vi "CHANGE_ITEM2STOCK.vi"(4 "date (to)":timestamp, 6 "date (From)":timestamp, 7 "connection reference":T1, 9 "DATABASE":string, 10 "data":T2[](array[typedef]), 11 "Output Type":string) -> (3 "Table Out":string[][](array[string]))   [LabVIEW 2015]
uses:
  Controls/ITEM_CODE_CLUSTER.ctl
  <vilib>/addons/database/Connection.llb/Conn ObjectReference.ctl
  <vilib>/addons/database/_DB Variant To Data/Database Variant To Data.xnode
  <vilib>/addons/database/NI_Database_API.lvlib
panel:
  in  "Data type":T2[](array[typedef])
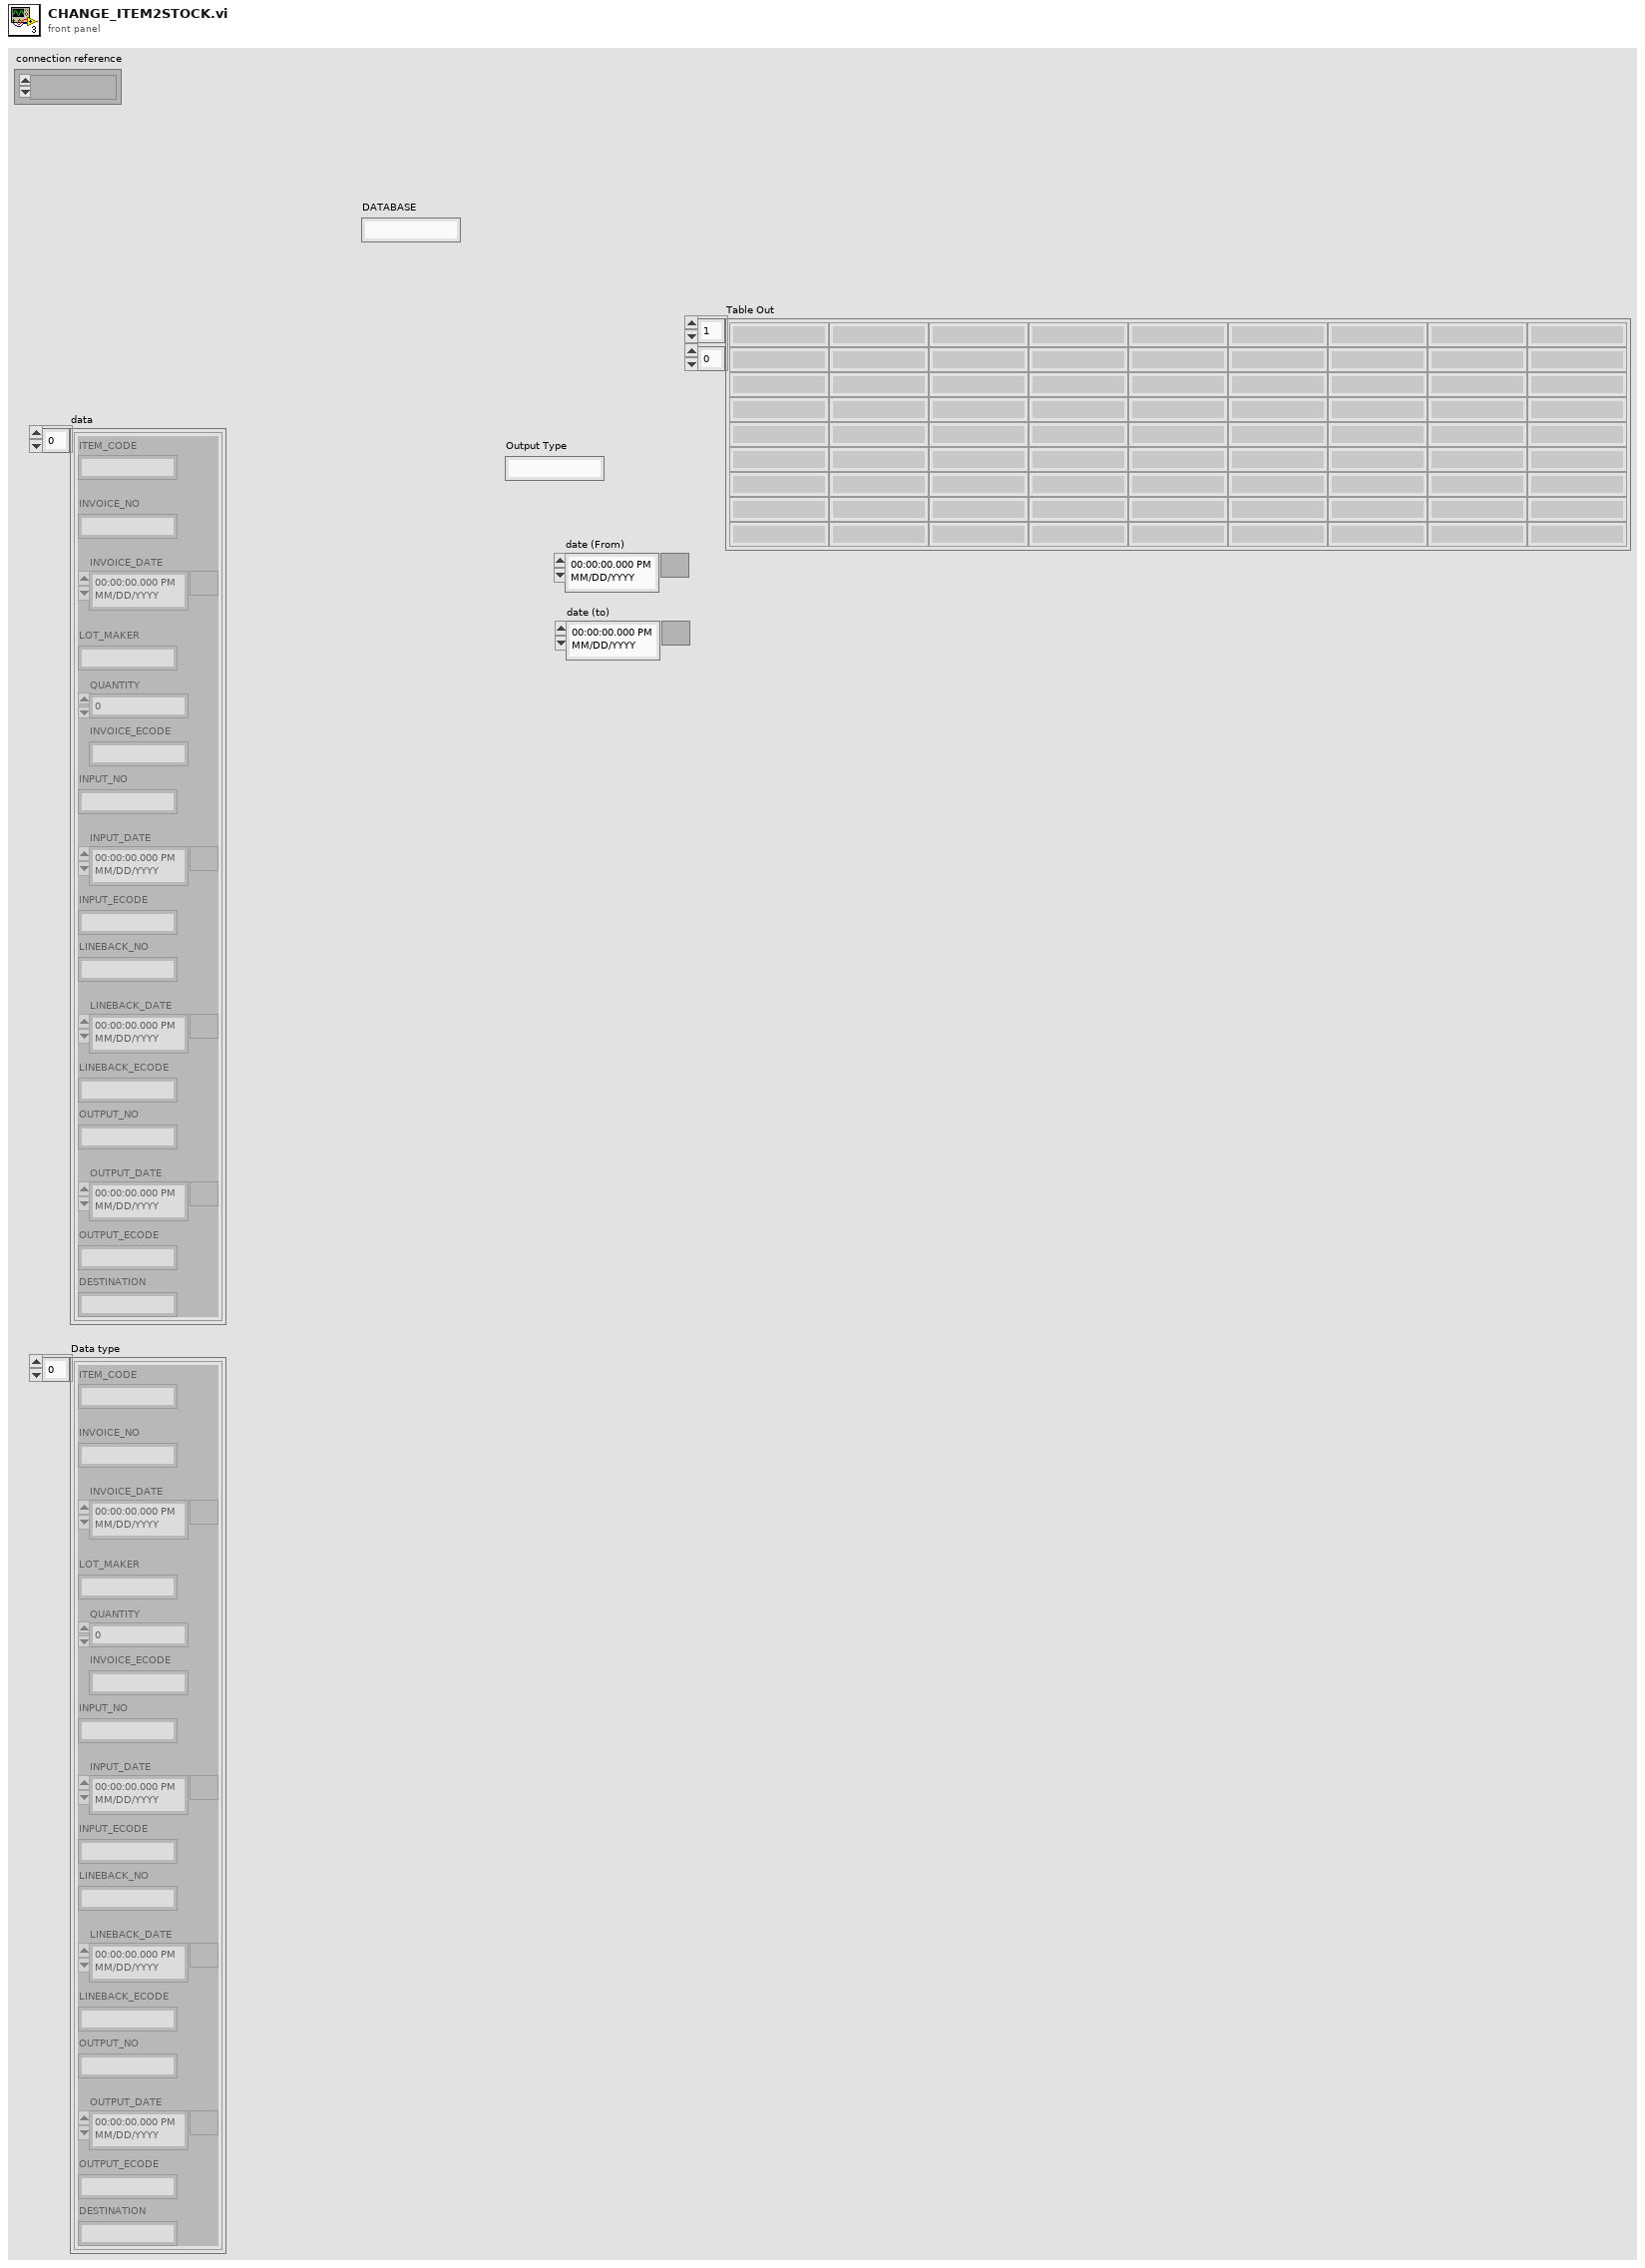
[diagram p1: front panel]
types:
  T1 = typedef "NI_Database_API.lvlib/Conn ObjectReference.ctl" = refnum<k1>
  T2 = typedef "ITEM_CODE_CLUSTER.ctl" = cluster{"ITEM_CODE":string, "INVOICE_NO":string, "INVOICE_DATE":timestamp, "LOT_MAKER":string, "QUANTITY":dbl, "INVOICE_ECODE":string, "INPUT_NO":string, "INPUT_DATE":timestamp, "INPUT_ECODE":string, "LINEBACK_NO":string, "LINEBACK_DATE":timestamp, "LINEBACK_ECODE":string, "OUTPUT_NO":string, "OUTPUT_DATE":timestamp, "OUTPUT_ECODE":string, "DESTINATION":string}
  T3 = cluster{"OUTPUT_DATE":timestamp, "Input":dbl, "Lineback":dbl, "QUANTITY":dbl, "Inline":dbl, "INVOICE_NO":string, "PO":string, "DESTINATION":string, "Stock":dbl, "Line Stock":dbl, "OUTPUT_ECODE":string, "PO":string}[]
  T4 = cluster{"LINEBACK_DATE":timestamp, "Input":dbl, "QUANTITY":dbl, "output":dbl, "Inline":dbl, "INVOICE_NO":string, "PO":string, "LINEBACK_NO":string, "Stock":dbl, "Line Stock":dbl, "LINEBACK_ECODE":string, "PO":string}[]
  T5 = cluster{"INPUT_DATE":timestamp, "QUANTITY":dbl, "Lineback":dbl, "output":dbl, "Inline":dbl, "INVOICE_NO":string, "PO":string, "Lot":string, "Stock":dbl, "Line Stock":dbl, "INPUT_ECODE":string, "INPUT_NO":string}[]
  T6 = cluster{"LINEBACK_DATE":timestamp, "Input":dbl, "QUANTITY":dbl, "output":dbl, "Inline":dbl, "INVOICE_NO":string, "PO":string, "LINEBACK_NO":string, "Stock":dbl, "Line Stock":dbl, "LINEBACK_ECODE":string, "PO":string}
  T7 = cluster{"OUTPUT_DATE":timestamp, "Input":dbl, "Lineback":dbl, "QUANTITY":dbl, "Inline":dbl, "INVOICE_NO":string, "OUTPUT_NO":string, "result string":string, "Stock":dbl, "Line Stock":dbl, "OUTPUT_ECODE":string, "PO":string}
  T8 = cluster{"INPUT_DATE":timestamp, "QUANTITY":dbl, "Lineback":dbl, "output":dbl, "Inline":dbl, "INVOICE_NO":string, "INPUT_NO":string, "Lot":string, "Stock":dbl, "Line Stock":dbl, "INPUT_ECODE":string, "INPUT_NO":string}
  T9 = cluster{"date (From)":timestamp, "input_initail":dbl, "line back initail":dbl, "output initail":dbl, "Inline":dbl, "PO":string, "PO":string, "PO":string, "Stock":dbl, "Line Stock":dbl, "PO":string, "PO":string}
  T10 = cluster{"INPUT_DATE":timestamp, "QUANTITY":dbl, "Lineback":dbl, "output":dbl, "Inline":dbl, "INVOICE_NO":string, "PO":string, "Lot":string, "Stock":dbl, "Line Stock":dbl, "INPUT_ECODE":string, "INPUT_NO":string}
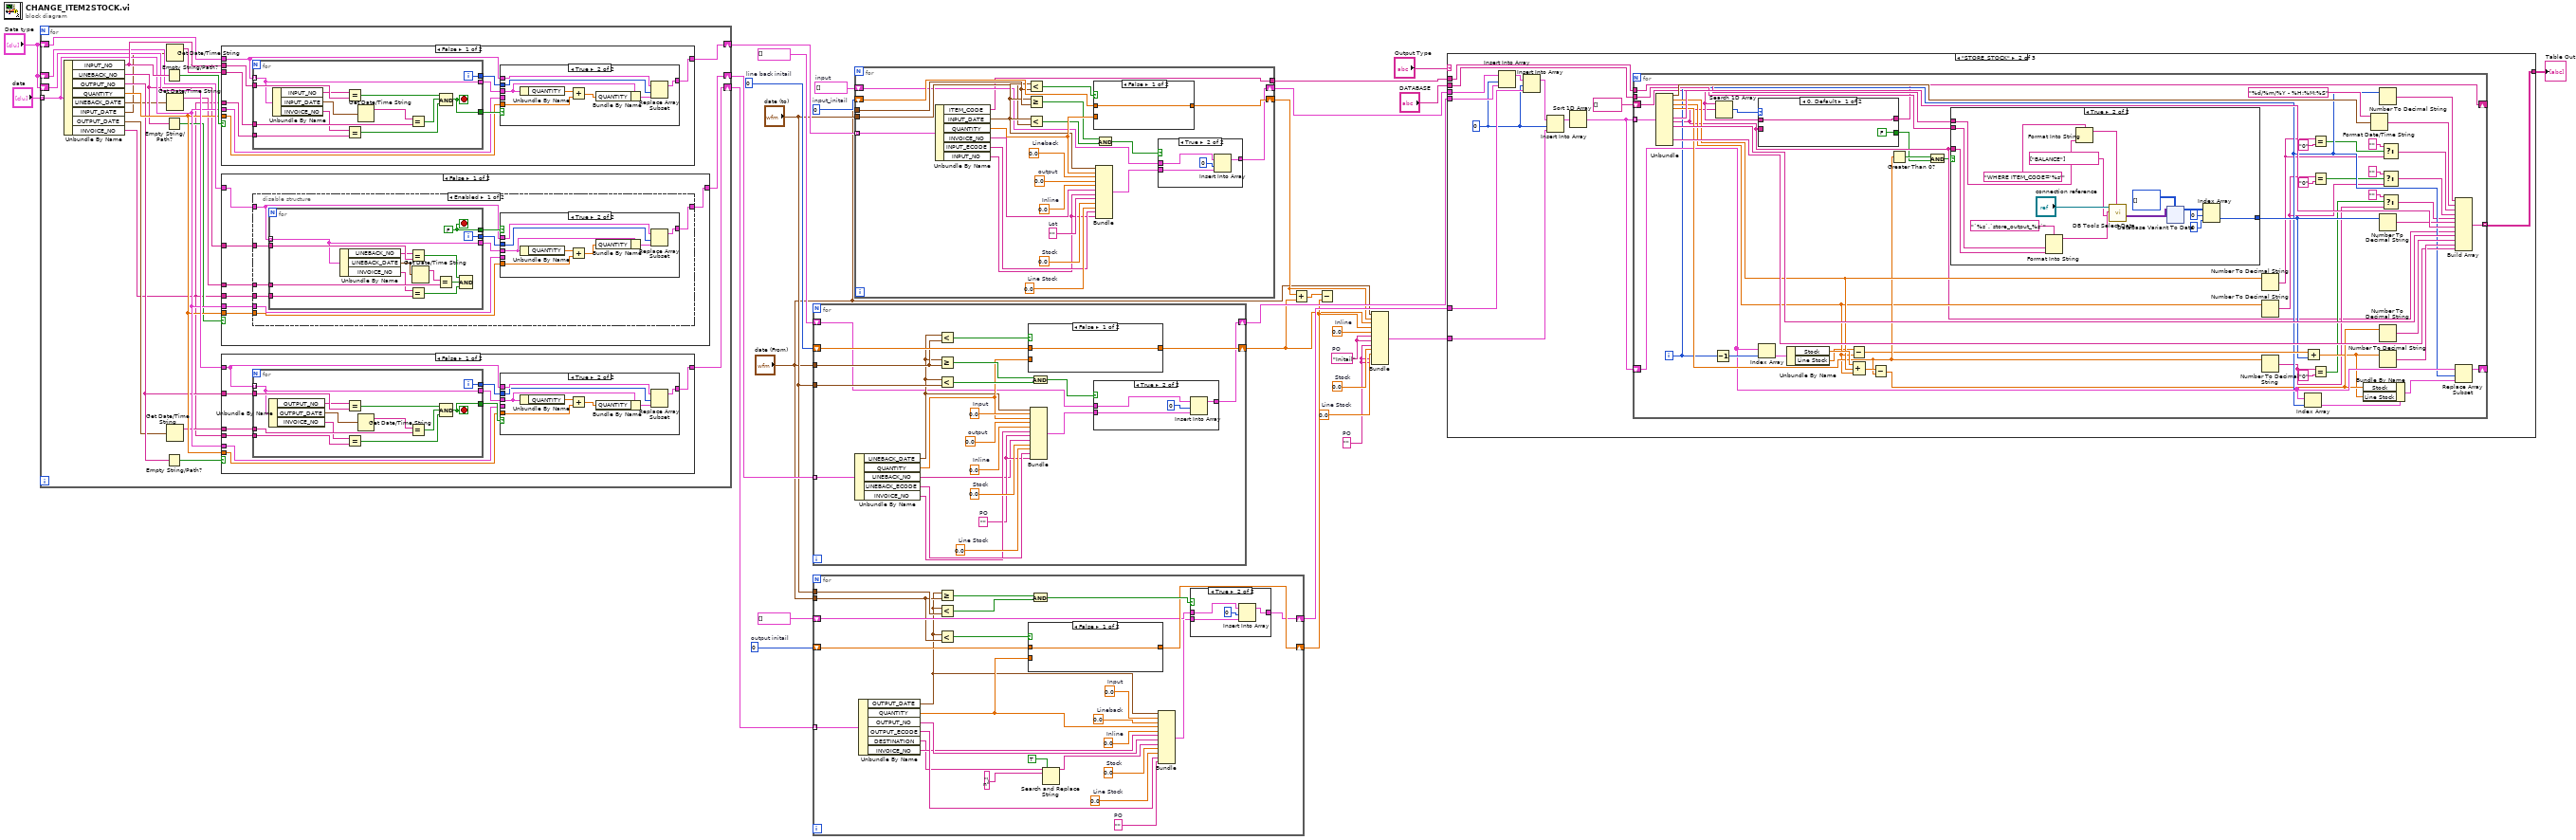
[diagram p0: block diagram]
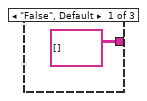
[diagram p2: hidden frame]
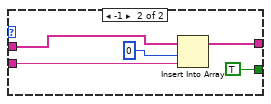
[diagram p3: hidden frame]
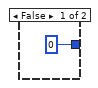
[diagram p4: hidden frame]
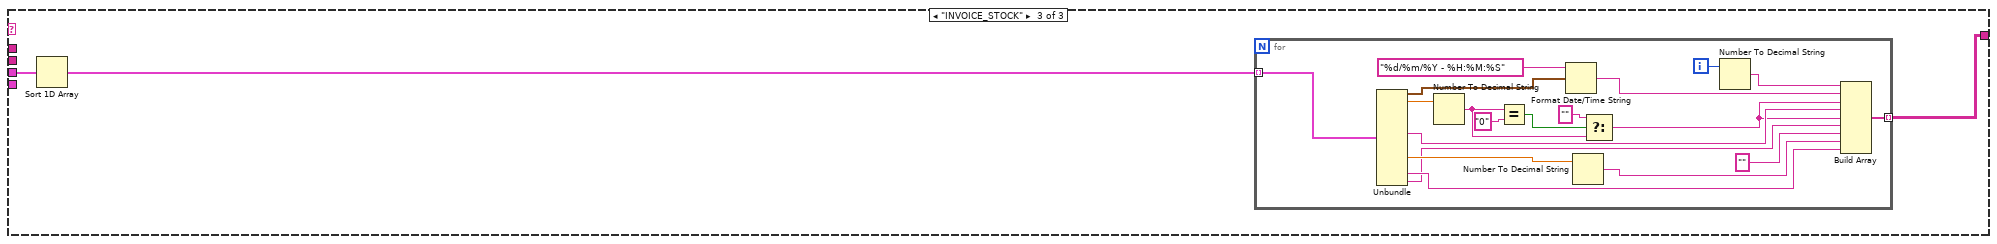
[diagram p5: hidden frame]
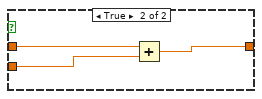
[diagram p7: hidden frame]
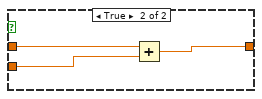
[diagram p9: hidden frame]
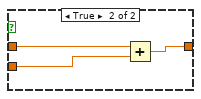
[diagram p11: hidden frame]
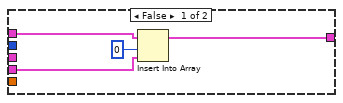
[diagram p12: hidden frame]
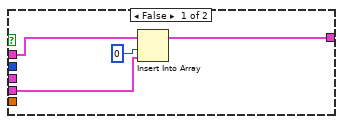
[diagram p14: hidden frame]
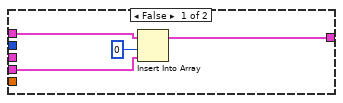
[diagram p17: hidden frame]
diagram:
  w5 = "Initail"  # PO
  w12 = 0.0  # Line Stock
  w11 = 0.0  # Stock
  w4 = ""  # PO
  w6 = 0.0  # Inline
  w17 = 0  # output initail
  w19 = 0  # line back initail
  w22 = T5 []  # input
  w23 = 0  # input_initail
  n1 = for {
    shift-right: [w48] -> w28
    shift-left: "Data type" -> [w51]
    shift-right: [w46] -> w29
    shift-left: "Data type" -> [w47]
    shift-right: [w44] -> w30
    shift-left: "Data type" -> [w45]
    tunnel: "data" -> [w43] mode=indexing
    n2 = Unbundle By Name(w43) -> ("INPUT_NO"=w50:string, "LINEBACK_NO"=w41:string, "OUTPUT_NO"=w39:string, "QUANTITY"=w42:dbl, "LINEBACK_DATE"=w37:timestamp, "INPUT_DATE"=w35:timestamp, "OUTPUT_DATE"=w33:timestamp, "INVOICE_NO"=w31:string)
    n3 = Empty String/Path?(string/path=w50) -> (empty?=w49:bool)
    n4 = Empty String/Path?(string/path=w41) -> (empty?=w40:bool)
    n5 = Empty String/Path?(string/path=w39) -> (empty?=w38:bool)
    n6 = Get Date/Time String(seconds (now)=w35) -> (date string=w34:string)  [unwired: 2 in, 1 out]
    n7 = Get Date/Time String(seconds (now)=w37) -> (date string=w36:string)  [unwired: 2 in, 1 out]
    n8 = Get Date/Time String(seconds (now)=w33) -> (date string=w32:string)  [unwired: 2 in, 1 out]
    n9 = case shown="False" w49 {
      tunnel: w51 -> [w138 w167]
      tunnel: w50 -> [w140 _]
      tunnel: w42 -> [w136 _]
      tunnel: [w135 w167] -> w48
      tunnel: w43 -> [w134 _]
      tunnel: w34 -> [w133 _]
      tunnel: w31 -> [w132 _]
      frame False {
        n10 = for {
          tunnel: w138 -> [w163] mode=indexing
          tunnel: w140 -> [w166]
          tunnel: [w157] -> w141
          tunnel: [w164] -> w139
          tunnel: [w163] -> w137
          tunnel: w133 -> [w162]
          tunnel: w132 -> [w156]
          i -> [w164]
          stop <- w157 stop-if-true
          n11 = Unbundle By Name(w163) -> ("INPUT_NO"=w165:string, "INPUT_DATE"=w161:timestamp, "INVOICE_NO"=w155:string)
          n12 = Equal?(x=w165, y=w166) -> (x = y?=w159:bool)
          n13 = Equal?(x=w155, y=w156) -> (x = y?=w154:bool)
          n14 = Get Date/Time String(seconds (now)=w161) -> (date string=w160:string)  [unwired: 2 in, 1 out]
          n15 = Equal?(x=w160, y=w162) -> (x = y?=w158:bool)
          n16 = Compound Arithmetic op=AND(w159, w158, w154) -> (w157:bool)
        }
        n17 = case shown="True" w141 {
          tunnel: w139 -> [_ w152]
          tunnel: w138 -> [w145 w153]
          tunnel: w137 -> [_ w150]
          tunnel: w136 -> [_ w148]
          tunnel: [w142 w147] -> w135
          tunnel: w134 -> [w144 _]
          frame False {
            n18 = Insert Into Array(array=w145, index=0, new element=w144) -> (w142:T2[])
          }
          frame True {
            n19 = Unbundle By Name(w150) -> ("QUANTITY"=w151:dbl)
            n20 = Add(x=w151, y=w148) -> (x+y=w149:dbl)
            n21 = Bundle By Name(cluster=w150, "QUANTITY"=w149) -> (w146:T2)
            n22 = Replace Array Subset(array=w153, new element=w146, index=w152) -> (w147:T2[])
          }
        }
      }
      frame True {
      }
    }
    n23 = case shown="False" w40 {
      tunnel: w47 -> [w93 w131]
      tunnel: w41 -> [w94 _]
      tunnel: w42 -> [w92 _]
      tunnel: [w91 w131] -> w46
      tunnel: w43 -> [w90 _]
      tunnel: w36 -> [w89 _]
      tunnel: w31 -> [w88 _]
      frame False {
        n24 = disable-structure shown="Enabled" {
          disable-tunnel: w94 -> [w103 _]
          disable-tunnel: w93 -> [w101 w130]
          disable-tunnel: w92 -> [w99 _]
          disable-tunnel: [w98 w130] -> w91
          disable-tunnel: w90 -> [w97 _]
          disable-tunnel: w89 -> [w96 _]
          disable-tunnel: w88 -> [w95 _]
          frame Enabled {
            n25 = for {
              tunnel: w101 -> [w126] mode=indexing
              tunnel: w103 -> [w129]
              tunnel: [w120] -> w104
              tunnel: [w127] -> w102
              tunnel: [w126] -> w100
              tunnel: w96 -> [w125]
              tunnel: w95 -> [w118]
              i -> [w127]
              stop <- w120 stop-if-true
              w120 = FALSE
              n26 = Unbundle By Name(w126) -> ("LINEBACK_NO"=w128:string, "LINEBACK_DATE"=w124:timestamp, "INVOICE_NO"=w119:string)
              n27 = Equal?(x=w128, y=w129) -> (x = y?=w122:bool)
              n28 = Equal?(x=w119, y=w118) -> (x = y?=w117:bool)
              n29 = Get Date/Time String(seconds (now)=w124) -> (date string=w123:string)  [unwired: 2 in, 1 out]
              n30 = Equal?(x=w123, y=w125) -> (x = y?=w121:bool)
              n31 = Compound Arithmetic op=AND(w122, w121, w117) -> ()  [unwired: 1 out]
            }
            n32 = case shown="True" w104 {
              tunnel: w102 -> [_ w115]
              tunnel: w101 -> [w108 w116]
              tunnel: w100 -> [_ w113]
              tunnel: w99 -> [_ w111]
              tunnel: [w105 w110] -> w98
              tunnel: w97 -> [w107 _]
              frame False {
                n33 = Insert Into Array(array=w108, index=0, new element=w107) -> (w105:T2[])
              }
              frame True {
                n34 = Unbundle By Name(w113) -> ("QUANTITY"=w114:dbl)
                n35 = Add(x=w114, y=w111) -> (x+y=w112:dbl)
                n36 = Bundle By Name(cluster=w113, "QUANTITY"=w112) -> (w109:T2)
                n37 = Replace Array Subset(array=w116, new element=w109, index=w115) -> (w110:T2[])
              }
            }
          }
          frame Disabled {
          }
        }
      }
      frame True {
      }
    }
    n38 = case shown="False" w38 {
      tunnel: w45 -> [w58 w87]
      tunnel: w39 -> [w60 _]
      tunnel: w42 -> [w56 _]
      tunnel: [w55 w87] -> w44
      tunnel: w43 -> [w54 _]
      tunnel: w32 -> [w53 _]
      tunnel: w31 -> [w52 _]
      frame False {
        n39 = for {
          tunnel: w58 -> [w83] mode=indexing
          tunnel: w60 -> [w86]
          tunnel: [w77] -> w61
          tunnel: [w84] -> w59
          tunnel: [w83] -> w57
          tunnel: w53 -> [w80]
          tunnel: w52 -> [w75]
          i -> [w84]
          stop <- w77 stop-if-true
          n40 = Unbundle By Name(w83) -> ("OUTPUT_NO"=w85:string, "OUTPUT_DATE"=w81:timestamp, "INVOICE_NO"=w76:string)
          n41 = Equal?(x=w85, y=w86) -> (x = y?=w79:bool)
          n42 = Equal?(x=w76, y=w75) -> (x = y?=w74:bool)
          n43 = Get Date/Time String(seconds (now)=w81) -> (date string=w82:string)  [unwired: 2 in, 1 out]
          n44 = Equal?(x=w82, y=w80) -> (x = y?=w78:bool)
          n45 = Compound Arithmetic op=AND(w79, w78, w74) -> (w77:bool)
        }
        n46 = case shown="True" w61 {
          tunnel: w59 -> [_ w72]
          tunnel: w58 -> [w65 w73]
          tunnel: w57 -> [_ w70]
          tunnel: w56 -> [_ w68]
          tunnel: [w62 w67] -> w55
          tunnel: w54 -> [w64 _]
          frame False {
            n47 = Insert Into Array(array=w65, index=0, new element=w64) -> (w62:T2[])
          }
          frame True {
            n48 = Unbundle By Name(w70) -> ("QUANTITY"=w71:dbl)
            n49 = Add(x=w71, y=w68) -> (x+y=w69:dbl)
            n50 = Bundle By Name(cluster=w70, "QUANTITY"=w69) -> (w66:T2)
            n51 = Replace Array Subset(array=w73, new element=w66, index=w72) -> (w67:T2[])
          }
        }
      }
      frame True {
      }
    }
  }
  n52 = for {
    tunnel: w29 -> [w190] mode=indexing
    tunnel: "date (From)" -> [w176]
    tunnel: "date (to)" -> [w177]
    shift-right: [w171] -> w18
    shift-left: T4 [] -> [w174]
    shift-right: [w172] -> w8
    shift-left: w19 -> [w179]
    w186 = 0.0  # Line Stock
    w187 = 0.0  # Stock
    w169 = ""  # PO
    w188 = 0.0  # Inline
    w189 = 0.0  # output
    w184 = 0.0  # Input
    n53 = Unbundle By Name(w190) -> ("LINEBACK_DATE"=w175:timestamp, "QUANTITY"=w178:dbl, "LINEBACK_NO"=w168:string, "LINEBACK_ECODE"=w185:string, "INVOICE_NO"=w170:string)
    n54 = Less?(x=w175, y=w176) -> (x < y?=w180:bool)
    n55 = Greater Or Equal?(x=w175, y=w176) -> (x >= y?=w181:bool)
    n56 = Less?(x=w175, y=w177) -> (x < y?=w182:bool)
    n57 = case shown="False" w180 {
      tunnel: w178 -> [_ w198]
      tunnel: w179 -> [w196 w199]
      tunnel: [w196 w197] -> w172
      frame False {
      }
      frame True {
        n58 = Add(x=w199, y=w198) -> (x+y=w197:dbl)
      }
    }
    n59 = Bundle("LINEBACK_DATE"=w175, "Input"=w184, "QUANTITY"=w178, "output"=w189, "Inline"=w188, "INVOICE_NO"=w170, "PO"=w169, "LINEBACK_NO"=w168, "Stock"=w187, "Line Stock"=w186, "LINEBACK_ECODE"=w185, "PO"=w169) -> (w173:T6)  [unwired: 1 in]
    n60 = And(x=w181, y=w182) -> (x .and. y?=w183:bool)
    n61 = case shown="True" w183 {
      tunnel: w174 -> [w191 w195]
      tunnel: w173 -> [_ w193]
      tunnel: [w191 w192] -> w171
      frame False {
      }
      frame True {
        n62 = Insert Into Array(array=w195, index=0, new element=w193) -> (w192:T4)
      }
    }
  }
  n63 = for {
    tunnel: w30 -> [w226] mode=indexing
    shift-right: [w213] -> w9
    shift-left: w17 -> [w215]
    shift-right: [w210] -> w14
    shift-left: T3 [] -> [w212]
    tunnel: "date (to)" -> [w209]
    tunnel: "date (From)" -> [w208]
    w223 = 0.0  # Line Stock
    w224 = 0.0  # Stock
    w205 = ""  # PO
    w225 = 0.0  # Inline
    w220 = 0.0  # Lineback
    w221 = 0.0  # Input
    n64 = Unbundle By Name(w226) -> ("OUTPUT_DATE"=w207:timestamp, "QUANTITY"=w214:dbl, "OUTPUT_NO"=w206:string, "OUTPUT_ECODE"=w222:string, "DESTINATION"=w202:string, "INVOICE_NO"=w204:string)
    n65 = Greater Or Equal?(x=w207, y=w208) -> (x >= y?=w217:bool)
    n66 = Less?(x=w207, y=w209) -> (x < y?=w218:bool)
    n67 = Less?(x=w207, y=w208) -> (x < y?=w216:bool)
    n68 = case shown="False" w216 {
      tunnel: w214 -> [_ w234]
      tunnel: w215 -> [w232 w235]
      tunnel: [w232 w233] -> w213
      frame False {
      }
      frame True {
        n69 = Add(x=w235, y=w234) -> (x+y=w233:dbl)
      }
    }
    n70 = And(x=w217, y=w218) -> (x .and. y?=w219:bool)
    n71 = Search and Replace String(replace all?=TRUE ("replace all? (F)"), input string=w202, search string="\n") -> (result string=w201:string)  [unwired: 5 in, 3 out]
    n72 = Bundle("OUTPUT_DATE"=w207, "Input"=w221, "Lineback"=w220, "QUANTITY"=w214, "Inline"=w225, "INVOICE_NO"=w204, "OUTPUT_NO"=w206, "result string"=w201, "Stock"=w224, "Line Stock"=w223, "OUTPUT_ECODE"=w222, "PO"=w205) -> (w211:T7)  [unwired: 1 in]
    n73 = case shown="True" w219 {
      tunnel: w212 -> [w227 w231]
      tunnel: w211 -> [_ w228]
      tunnel: [w227 w229] -> w210
      frame False {
      }
      frame True {
        n74 = Insert Into Array(array=w231, index=0, new element=w228) -> (w229:T3)
      }
    }
  }
  n75 = for {
    tunnel: w28 -> [w259] mode=indexing
    tunnel: "date (From)" -> [w246]
    tunnel: "date (to)" -> [w244]
    shift-right: [w247] -> w10
    shift-left: w23 -> [w248]
    shift-right: [w238] -> w21
    shift-left: w22 -> [w240]
    tunnel: [w237] -> w1
    w252 = 0.0  # Line Stock
    w253 = 0.0  # Stock
    w254 = ""  # Lot
    w256 = 0.0  # Inline
    w257 = 0.0  # output
    w258 = 0.0  # Lineback
    n76 = Unbundle By Name(w259) -> ("ITEM_CODE"=w237:string, "INPUT_DATE"=w245:timestamp, "QUANTITY"=w249:dbl, "INVOICE_NO"=w255:string, "INPUT_ECODE"=w251:string, "INPUT_NO"=w236:string)
    n77 = Less?(x=w245, y=w246) -> (x < y?=w250:bool)
    n78 = Greater Or Equal?(x=w245, y=w246) -> (x >= y?=w243:bool)
    n79 = Less?(x=w245, y=w244) -> (x < y?=w242:bool)
    n80 = case shown="False" w250 {
      tunnel: w249 -> [_ w267]
      tunnel: w248 -> [w265 w268]
      tunnel: [w265 w266] -> w247
      frame False {
      }
      frame True {
        n81 = Add(x=w268, y=w267) -> (x+y=w266:dbl)
      }
    }
    n82 = Bundle("INPUT_DATE"=w245, "QUANTITY"=w249, "Lineback"=w258, "output"=w257, "Inline"=w256, "INVOICE_NO"=w255, "INPUT_NO"=w236, "Lot"=w254, "Stock"=w253, "Line Stock"=w252, "INPUT_ECODE"=w251, "INPUT_NO"=w236) -> (w239:T8)  [unwired: 1 in]
    n83 = And(x=w243, y=w242) -> (x .and. y?=w241:bool)
    n84 = case shown="True" w241 {
      tunnel: w240 -> [w260 w264]
      tunnel: w239 -> [_ w262]
      tunnel: [w260 w261] -> w238
      frame False {
      }
      frame True {
        n85 = Insert Into Array(array=w264, index=0, new element=w262) -> (w261:T5)
      }
    }
  }
  n86 = Add(x=w10, y=w8) -> (x+y=w13:dbl)
  n87 = Subtract(x=w13, y=w9) -> ()  [unwired: 1 out]
  n88 = Bundle("date (From)"="date (From)", "input_initail"=w10, "line back initail"=w8, "output initail"=w9, "Inline"=w6, "PO"=w5, "PO"=w5, "PO"=w4, "Stock"=w11, "Line Stock"=w12, "PO"=w4, "PO"=w4) -> (w3:T9)  [unwired: 1 in]
  n89 = case shown="\"STORE_STOCK\"" "Output Type" {
    tunnel: w14 -> [_ w282 _]
    tunnel: w18 -> [_ w280 _]
    tunnel: w21 -> [_ w279 w403]
    tunnel: [string[][] [] w278 w404] -> w25
    tunnel: w3 -> [_ w274 _]
    tunnel: "DATABASE" -> [_ w272 _]
    tunnel: w1 -> [_ w271 _]
    frame "False", Default {
    }
    frame "STORE_STOCK" {
      w276 = 0 ("index")
      n90 = Insert Into Array(array=w279, index=w276, new element=w280) -> (w281:T5)
      n91 = Insert Into Array(array=w281, index=w276, new element=w282) -> (w277:T5)
      n92 = Insert Into Array(array=w277, index=w276, new element=w274) -> (w275:T5)
      n93 = Sort 1D Array(array=w275) -> (sorted array=w273:T5)
      n94 = for {
        tunnel: w273 -> [w335] mode=indexing
        tunnel: [w325] -> w278 mode=indexing
        tunnel: w272 -> [w324]
        tunnel: w271 -> [w323]
        shift-right: [w305] -> _
        shift-left: w273 -> [w310]
        shift-right: [w286] -> _
        shift-left: string[] [] -> [w288]
        i -> [w309]
        n95 = Unbundle(w335) -> ("INPUT_DATE"=w334:timestamp, "QUANTITY"=w319:dbl, "Lineback"=w316:dbl, "output"=w317:dbl, "INVOICE_NO"=w330:string, "PO"=w287:string, "Lot"=w329:string, "INPUT_ECODE"=w326:string)  [unwired: 4 out]
        n96 = Decrement(x=w309) -> (x-1=w322:i32)
        n97 = Search 1D Array(1D array=w288, element=w287) -> (index of element=w289:i32)  [unwired: 1 in]
        n98 = case shown="0, Default" w289 {
          tunnel: w288 -> [w337 w342]
          tunnel: w287 -> [_ w341]
          tunnel: [w337 w339] -> w286
          tunnel: [FALSE TRUE] -> w284
          frame 0, Default {
          }
          frame -1 {
            n99 = Insert Into Array(array=w342, index=0, new element=w341) -> (w339:string[])
          }
        }
        n100 = Index Array(array=w310, index=w322) -> (element=w321:T10)
        n101 = Unbundle By Name(w321) -> ("Stock"=w320:dbl, "Line Stock"=w312:dbl)
        n102 = Subtract(x=w312, y=w316) -> (x-y=w315:dbl)
        n103 = Compound Arithmetic op=ADD(w320, w319, w316) -> (w318:dbl)
        n104 = Subtract(x=w318, y=w317) -> (x-y=w308:dbl)
        n105 = Greater Than 0?(x=w317) -> (x > 0?=w285:bool)
        n106 = And(x=w285, y=w284) -> (x .and. y?=w283:bool)
        n107 = case shown="True" w283 {
          tunnel: w324 -> [_ w356]
          tunnel: w287 -> [_ w355]
          tunnel: w323 -> [_ w351]
          tunnel: [0 w344] -> w313
          frame False {
          }
          frame True {
            n108 = Format Into String(format string="`%s`.`store_output_%s`", w356, w355) -> (resulting string=w354:string)  [unwired: 2 in, 1 out]
            n109 = Format Into String(format string="WHERE ITEM_CODE='%s'" ("condition"), w351) -> (resulting string=w350:string)  [unwired: 2 in, 1 out]
            n110 = call <vilib>:"DB Tools Select Data.vi"("condition"=w350, "columns"=string[] ["BALANCE"], "table"=w354, "connection reference"="connection reference") -> ("data"=w349:variant[][])  [unwired: 2 in, 2 out]
            n111 = xnode "Database Variant To Data"("database variant"=w349, "type"=i32[][] []) -> ("data"=w345:i32[][])  [unwired: 1 in, 1 out]
            n112 = Index Array(array=w345, index (row)=0, index (col)=0 ("disabled index (col)")) -> (element=w344:i32)
          }
        }
        n113 = Number To Decimal String(number=w319) -> (decimal integer string=w300:string)  [unwired: 1 in]
        n114 = Number To Decimal String(number=w316) -> (decimal integer string=w296:string)  [unwired: 1 in]
        n115 = Number To Decimal String(number=w317) -> (decimal integer string=w291:string)  [unwired: 1 in]
        n116 = Index Array(array=w310, index=w309) -> (element=w311:T10)
        n117 = Add(x=w315, y=w313) -> (x+y=w307:dbl)
        n118 = Equal?(x=w300, y="0") -> (x = y?=w303:bool)
        n119 = Equal?(x=w296, y="0") -> (x = y?=w298:bool)
        n120 = Equal?(x=w291, y="0") -> (x = y?=w293:bool)
        n121 = Bundle By Name(cluster=w311, "Stock"=w308, "Line Stock"=w307) -> (w306:T10)
        n122 = Format Date/Time String(time format string (%c)="%d/%m/%Y - %H:%M:%S", seconds (now)=w334) -> (date/time string=w331:string)  [unwired: 1 in]
        n123 = Number To Decimal String(number=w309) -> (decimal integer string=w332:string)  [unwired: 1 in]
        n124 = Number To Decimal String(number=w313) -> (decimal integer string=w314:string)  [unwired: 1 in]
        n125 = Number To Decimal String(number=w308) -> (decimal integer string=w328:string)  [unwired: 1 in]
        n126 = Number To Decimal String(number=w307) -> (decimal integer string=w327:string)  [unwired: 1 in]
        n127 = Select(t="" ("y"), s=w303, f=w300) -> (s? t:f=w302:string)
        n128 = Select(t="" ("y"), s=w298, f=w296) -> (s? t:f=w295:string)
        n129 = Select(t="" ("y"), s=w293, f=w291) -> (s? t:f=w290:string)
        n130 = Build Array(w332, w331, w302, w295, w290, w314, w330, w287, w329, w328, w327, w326) -> (w325:string[])
        n131 = Replace Array Subset(array=w310, new element=w306, index=w309) -> (w305:T5)
      }
    }
    frame "INVOICE_STOCK" {
      n132 = Sort 1D Array(array=w403) -> (sorted array=w405:T5)
      n133 = for {
        tunnel: w405 -> [w424] mode=indexing
        tunnel: [w416] -> w404 mode=indexing
        i -> [w421]
        n134 = Unbundle(w424) -> ("INPUT_DATE"=w423:timestamp, "QUANTITY"=w418:dbl, "INVOICE_NO"=w415:string, "Stock"=w414:dbl, "INPUT_ECODE"=w417:string, "INPUT_NO"=w411:string)  [unwired: 6 out]
        n135 = Number To Decimal String(number=w418) -> (decimal integer string=w407:string)  [unwired: 1 in]
        n136 = Equal?(x=w407, y="0") -> (x = y?=w409:bool)
        n137 = Format Date/Time String(time format string (%c)="%d/%m/%Y - %H:%M:%S", seconds (now)=w423) -> (date/time string=w419:string)  [unwired: 1 in]
        n138 = Number To Decimal String(number=w414) -> (decimal integer string=w413:string)  [unwired: 1 in]
        n139 = Select(t="" ("y"), s=w409, f=w407) -> (s? t:f=w406:string)
        n140 = Number To Decimal String(number=w421) -> (decimal integer string=w420:string)  [unwired: 1 in]
        n141 = Build Array(w420, w419, w406, w415, w406, w411, "" ("element"), w413, w417) -> (w416:string[])
      }
    }
  }
  "Table Out" <- w25
